vi "PLC_InitialExcel.vi"(11 "Tbl引用句柄":refnum<vi>) -> ()   [LabVIEW 2017]
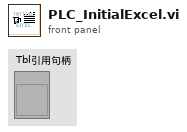
[diagram p1: front panel]
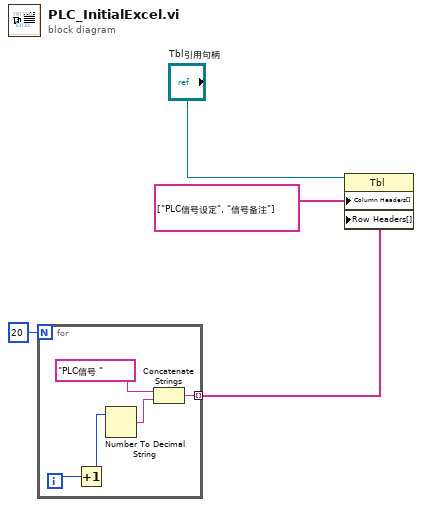
[diagram p0: block diagram]
diagram:
  n1 = for {
    N: 20 -> [_]
    tunnel: [w5] -> w1 mode=indexing
    i -> [w9]
    n2 = Increment(x=w9) -> (x+1=w7:i32)
    n3 = Number To Decimal String(number=w7) -> (decimal integer string=w6:string)  [unwired: 1 in]
    n4 = Concatenate Strings("PLC信号 ", w6) -> (w5:string)
  }
  n5 = property class="Tbl"(reference="Tbl引用句柄", "Column Headers[]"=string[] ["PLC信号设定", "信号备注"] ("列首字符串[]"), "Row Headers[]"=w1) -> ()  [unwired: 1 in, 2 out]
